vi "Teleop.vi"(10 "Match Info":T1={"Autonomous Elapsed Seconds"=0.0, "TeleOp Elapsed Seconds"=0.0, "Disabled Elapsed Seconds"=0.0, "Visited Autonomous"=FALSE, "Visited TeleOp"=FALSE, "Visited Disabled"=FALSE, "Autonomous Settings"={"Autonomous Style"=enum."Independent", "VI Refnum"=refnum}}, 11 "Call Context":T2) -> ()   [LabVIEW 2014]
doc: "This VI is called for each TeleOp packet received from the DS where the robot is not disabled. It is often used to read from the joysticks and update I/O or to update setpoints for timed control loops. It should complete and return within 20 milliseconds or it may miss DS packets."
uses:
  <vilib>/Rock Robotics/WPI/DriverStation/WPI_DriverStationDerivedRobotMode.ctl
  <vilib>/Rock Robotics/WPI/DriverStation/WPI_DriverStationMatch Info.ctl
  <vilib>/Rock Robotics/WPI/RobotDrive/WPI_RobotDriveGetSetRefNum.vi
  <vilib>/Rock Robotics/WPI/Joystick/WPI_JoystickGetSetRefNum.vi
  <vilib>/Rock Robotics/Network Tables/SD Write Boolean Array.vi
  <vilib>/Rock Robotics/Network Tables/SD Write Numeric Array.vi
  <vilib>/Rock Robotics/Network Tables/SD Write Number.vi
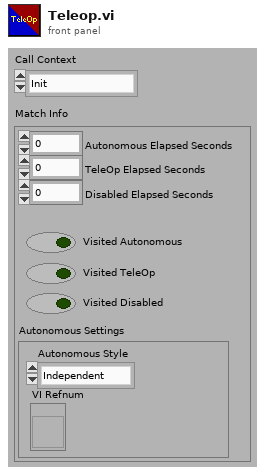
[diagram p1: front panel]
types:
  T1 = typedef "WPI_DriverStationMatch Info.ctl" = cluster{"Autonomous Elapsed Seconds":dbl, "TeleOp Elapsed Seconds":dbl, "Disabled Elapsed Seconds":dbl, "Visited Autonomous":bool, "Visited TeleOp":bool, "Visited Disabled":bool, "Autonomous Settings":cluster{"Autonomous Style":enum16{"Iterative", "Independent"}, "VI Refnum":refnum<vi>}}
  T2 = typedef "WPI_DriverStationDerivedRobotMode.ctl" = enum16{"Init", "Execute", "Stop"}
  T3 = typedef "WPI_JoystickDevRef.ctl" = cluster{"Device":T4}
  T4 = typedef "WPI_JoystickDeviceEnum.ctl" = enum16{"USB 0", "USB 1", "USB 2", "USB 3", "USB 4", "USB 5"}
  T5 = typedef "WPI_MotorControlDeviceRef.ctl" = cluster{"DeviceStatus":errorcluster, "Type":T6, "PWM":cluster{"Controller":T7, "PWM Channel":T8, "DeadBand":T9}, "CAN":cluster{"Device Number":u8, "Control Mode":T10, "Semaphore":T11, "Max Vout":dbl, "TalonSRX Control Mode":T12}, "Invert":bool, "TransformRef":T13, "InvTransformRef":T13}
  T6 = typedef "WPI_MotorControlType.ctl" = enum16{"PWM", "CAN", "CANTalonSRX"}
  T7 = typedef "FPGA_TypedefDigitalModule.ctl" = enum16{"Controller 1"}
  T8 = typedef "FPGA_DIOPWMChannel.ctl" = enum8{"PWM 0", "PWM 1", "PWM 2", "PWM 3", "PWM 4", "PWM 5", "PWM 6", "PWM 7", "PWM 8", "PWM 9", "PWM MXP 0", "PWM MXP 1", "PWM MXP 2", "PWM MXP 3", "PWM MXP 4", "PWM MXP 5", "PWM MXP 6", "PWM MXP 7", "PWM MXP 8", "PWM MXP 9", "Invalid"}
  T9 = typedef "WPI_PWMDeadband.ctl" = cluster{"Name":string, "maxPositivePwm":i32, "minPositivePwm":i32, "centerPwm":i32, "maxNegativePwm":i32, "minNegativePwm":i32, "angularRange":u16}
  T10 = typedef "WPI_CANJaguar_ControlMode.ctl" = enum8{"Percent VBus", "Current", "Speed", "Position", "Voltage"}
  T11 = typedef "Semaphore RefNum" = refnum<k1>
  T12 = typedef "WPI_CANTalonSRX_APIControlMode.ctl" = enum8{"Percent VBus", "Speed", "Position", "Slave", "Unchanged / Invalid"}
  T13 = typedef "WPI_PWMTransform_ConPane.ctl" = refnum<vi>
  T14 = typedef "WPI_RobotDriveDevRef.ctl" = cluster{"DevStatus":errorcluster, "Motors[]":T5[], "Square Inputs":bool, "Max Output":dbl}
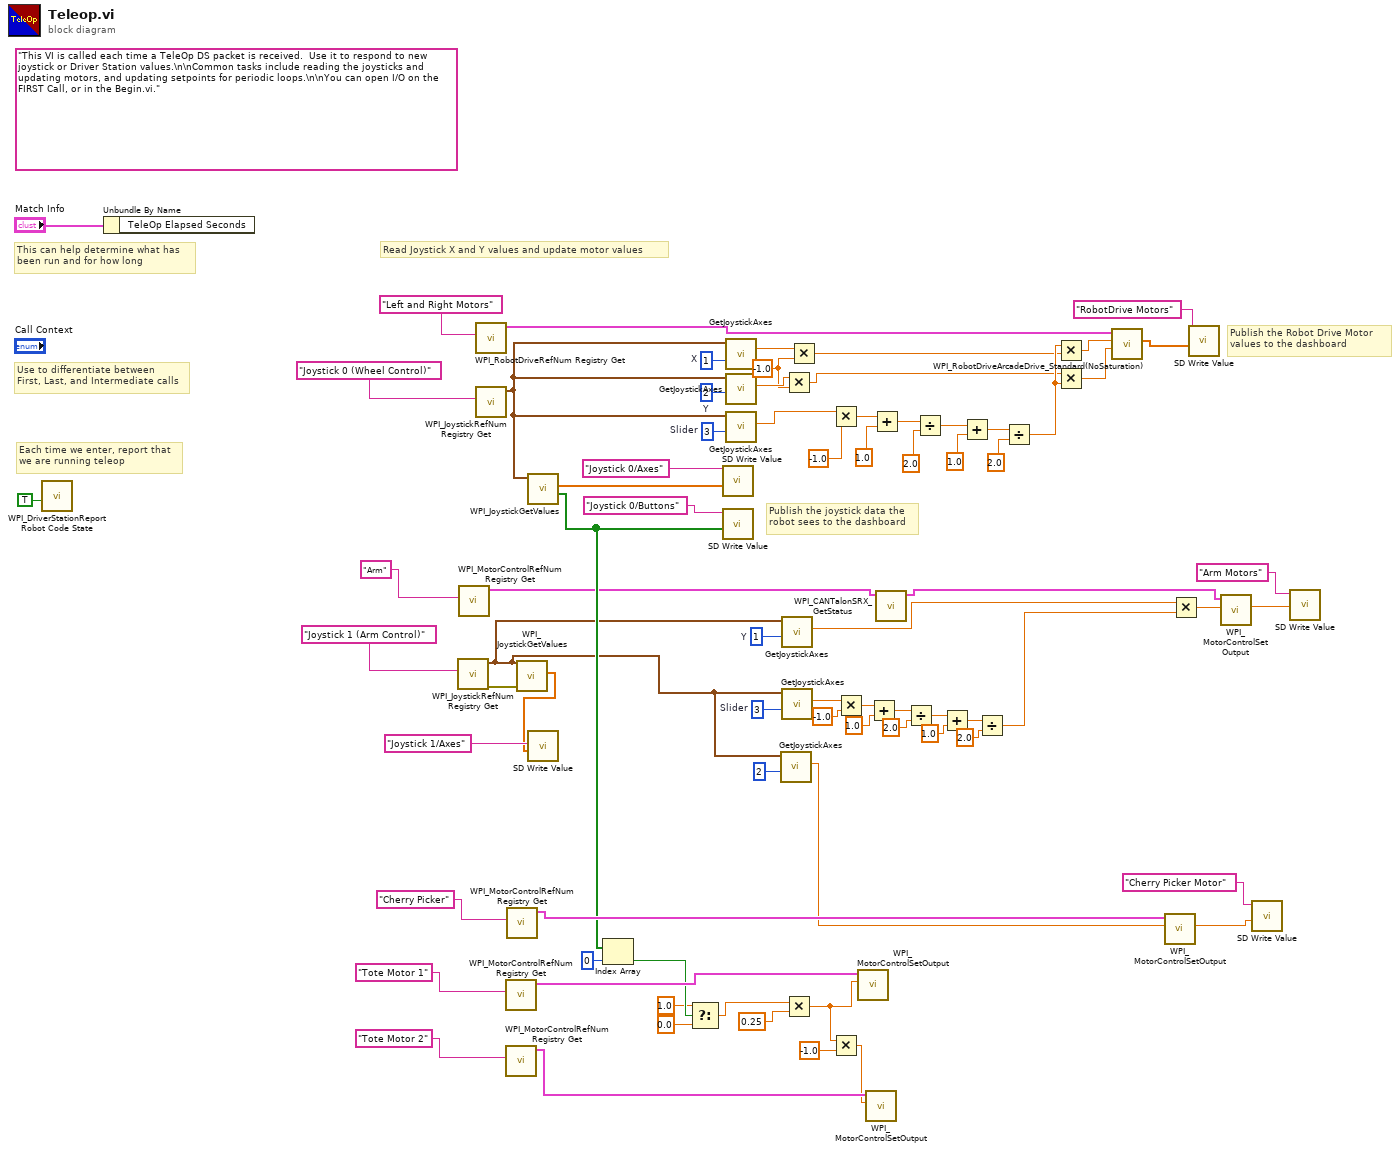
[diagram p0: block diagram]
diagram:
  w2 = -1.0 ("y")
  w10 = 3  # Slider
  w12 = 1  # Y
  w16 = 2  # Y
  w17 = 1  # X
  w14 = 3  # Slider
  (unwired) "This VI is called each time a TeleOp DS packet is received.  Use it to respond to new joystick or Driver Station values.\n\nCommon tasks include reading the joysticks and updating motors, and updating setpoints for periodic loops.\n\nYou can open I/O on the FIRST Call, or in the Begin.vi."
  # "Publish the Robot Drive Motor\nvalues to the dashboard"
  # "Publish the joystick data the\nrobot sees to the dashboard"
  # "Each time we enter, report that\nwe are running teleop"
  # "Use to differentiate between\nFirst, Last, and Intermediate calls"
  # "This can help determine what has\nbeen run and for how long"
  # "Read Joystick X and Y values and update motor values"
  n1 = call <vilib>:"WPI_DriverStationReport Robot Code State.vi"("TeleOp"=TRUE ("Autonomous")) -> ()  [unwired: 10 in, 1 out]
  n2 = Unbundle By Name("Match Info") -> ()  [unwired: 1 out]
  n3 = call <vilib>:"WPI_JoystickRefNum Registry Get.vi"("refnum name"="Joystick 1 (Arm Control)") -> ("error out"=w53:errorcluster, "JoystickDevRef"=w8:T3)  [unwired: 1 in, 8 out]
  n4 = call <vilib>:"WPI_MotorControlRefNum Registry Get.vi"("refnum name"="Arm") -> ("MotorControlDevRef"=w22:T5)  [unwired: 9 in, 1 out]
  n5 = call <vilib>:"WPI_RobotDriveRefNum Registry Get.vi"("refnum name"="Left and Right Motors") -> ("RobotDriveDevRef"=w75:T14)  [unwired: 1 in, 9 out]
  n6 = call <vilib>:"WPI_JoystickRefNum Registry Get.vi"("refnum name"="Joystick 0 (Wheel Control)") -> ("JoystickDevRef"=w15:T3)  [unwired: 1 in, 9 out]
  n7 = call <vilib>:"WPI_MotorControlRefNum Registry Get.vi"("refnum name"="Tote Motor 1") -> ("MotorControlDevRef"=w35:T5)  [unwired: 9 in, 1 out]
  n8 = call <vilib>:"WPI_MotorControlRefNum Registry Get.vi"("refnum name"="Tote Motor 2") -> ("MotorControlDevRef"=w34:T5)  [unwired: 9 in, 1 out]
  n9 = call <vilib>:"WPI_MotorControlRefNum Registry Get.vi"("refnum name"="Cherry Picker") -> ("MotorControlDevRef"=w41:T5)  [unwired: 9 in, 1 out]
  n10 = call <vilib>:"WPI_JoystickGetValues.vi"("error in (no error)"=w53, "JoystickDevRef"=w8) -> ("Axes"=w42:dbl[])  [unwired: 5 in, 4 out]
  n11 = call <vilib>:"WPI_JoystickGetValues.vi"("JoystickDevRef"=w15) -> ("Buttons"=w30:bool[], "Axes"=w33:dbl[])  [unwired: 6 in, 3 out]
  n12 = call-poly <vilib>:"SD Write Value.vi"("Numeric Array"=w42, "Name"="Joystick 1/Axes") -> ()  [unwired: 8 in, 2 out]
  n13 = Index Array(array=w30, index=0) -> (element=w29:bool)
  n14 = Select(t=1.0, s=w29, f=0.0) -> (s? t:f=w26:dbl)
  n15 = call-poly <vilib>:"SD Write Value.vi"("Numeric Array"=w33, "Name"="Joystick 0/Axes") -> ()  [unwired: 8 in, 2 out]
  n16 = call-poly <vilib>:"SD Write Value.vi"("Boolean Array"=w30, "Name"="Joystick 0/Buttons") -> ()  [unwired: 8 in, 2 out]
  n17 = call "GetJoystickAxes.vi"("Axes ID"=w17, "JoystickDevRef"=w15) -> ("element"=w3:dbl)  [unwired: 9 in]
  n18 = call "GetJoystickAxes.vi"("Axes ID"=w16, "JoystickDevRef"=w15) -> ("element"=w5:dbl)  [unwired: 9 in]
  n19 = call "GetJoystickAxes.vi"("Axes ID"=w14, "JoystickDevRef"=w15) -> ("element"=w13:dbl)  [unwired: 9 in]
  n20 = call "GetJoystickAxes.vi"("Axes ID"=2 ("index"), "JoystickDevRef"=w8) -> ("element"=w6:dbl)  [unwired: 9 in]
  n21 = call "GetJoystickAxes.vi"("Axes ID"=w12, "JoystickDevRef"=w8) -> ("element"=w11:dbl)  [unwired: 9 in]
  n22 = call "GetJoystickAxes.vi"("Axes ID"=w10, "JoystickDevRef"=w8) -> ("element"=w9:dbl)  [unwired: 9 in]
  n23 = Multiply(x=w5, y=w2) -> (x*y=w4:dbl)
  n24 = Multiply(x=w26, y=0.25) -> (x*y=w25:dbl)
  n25 = Multiply(x=w3, y=w2) -> (x*y=w1:dbl)
  n26 = Multiply(x=w13, y=-1.0 ("x")) -> (x*y=w56:dbl)
  n27 = Multiply(x=w25, y=-1.0) -> (x*y=w24:dbl)
  n28 = Multiply(x=w9, y=-1.0 ("x")) -> (x*y=w45:dbl)
  n29 = call <vilib>:"WPI_MotorControlSetOutput.vi"("Output"=w25, "MotorControlDevRef"=w35) -> ()  [unwired: 7 in, 3 out]
  n30 = call <vilib>:"WPI_MotorControlSetOutput.vi"("Output"=w24, "MotorControlDevRef"=w34) -> ()  [unwired: 7 in, 3 out]
  n31 = Add(x=w45, y=1.0 ("x")) -> (x+y=w52:dbl)
  n32 = Add(x=w56, y=1.0 ("x")) -> (x+y=w68:dbl)
  n33 = call <vilib>:"WPI_CANTalonSRX_GetStatus.vi"("CAN Talon SRX Ref"=w22) -> ("CAN Talon SRX Ref Out"=w18:T5)  [unwired: 8 in, 2 out]
  n34 = Divide(x=w52, y=2.0 ("x")) -> (x/y=w49:dbl)
  n35 = Divide(x=w68, y=2.0 ("x")) -> (x/y=w61:dbl)
  n36 = Add(x=w49, y=1.0) -> (x+y=w48:dbl)
  n37 = Add(x=w61, y=1.0) -> (x+y=w60:dbl)
  n38 = Divide(x=w48, y=2.0) -> (x/y=w43:dbl)
  n39 = Divide(x=w60, y=2.0) -> (x/y=w58:dbl)
  n40 = Multiply(x=w58, y=w1) -> (x*y=w65:dbl)
  n41 = Multiply(x=w4, y=w58) -> (x*y=w66:dbl)
  n42 = call <vilib>:"WPI_RobotDriveArcadeDrive_Standard(NoSaturation).vi"("Y axis value"=w66, "X axis value"=w65, "RobotDriveDevRef"=w75) -> ("Motor Values"=w71:dbl[])  [unwired: 1 in, 7 out]
  n43 = call <vilib>:"WPI_MotorControlSetOutput.vi"("Output"=w6, "MotorControlDevRef"=w41) -> ("Motor Output"=w39:dbl)  [unwired: 7 in, 2 out]
  n44 = Multiply(x=w11, y=w43) -> (x*y=w19:dbl)
  n45 = call-poly <vilib>:"SD Write Value.vi"("Numeric Array"=w71, "Name"="RobotDrive Motors") -> ()  [unwired: 8 in, 2 out]
  n46 = call <vilib>:"WPI_MotorControlSetOutput.vi"("Output"=w19, "MotorControlDevRef"=w18) -> ("Motor Output"=w20:dbl)  [unwired: 7 in, 2 out]
  n47 = call-poly <vilib>:"SD Write Value.vi"("Numeric"=w39, "Name"="Cherry Picker Motor") -> ()  [unwired: 8 in, 2 out]
  n48 = call-poly <vilib>:"SD Write Value.vi"("Numeric"=w20, "Name"="Arm Motors") -> ()  [unwired: 8 in, 2 out]
